vi "Ins_UARTWithBuffer.vi"(0 "COM":refnum<visa-resource-name>, 1 "Send":string, 3 "Timeout (ms)":u32=2000, 5 "Function":T1(ring)=enum."SendCompare", 9 "Baudrate":u32=921600, 11 "error in (no error)":errorcluster, 12 "REC":string) -> (6 "pass?":bool, 8 "ReceiveString":string, 10 "Return":string, 15 "error out":errorcluster)   [LabVIEW 2020, in "UART.lvlib"]
uses:
  UART.lvlib
  <vilib>/Instr/_visa.llb/VISA Set IO Buffer Mask.ctl
  75df8ced-9b69-4a5e-8517-458ef4cbff5d.vi
  <vilib>/Instr/_visa.llb/VISA Configure Serial Port (Instr).vi
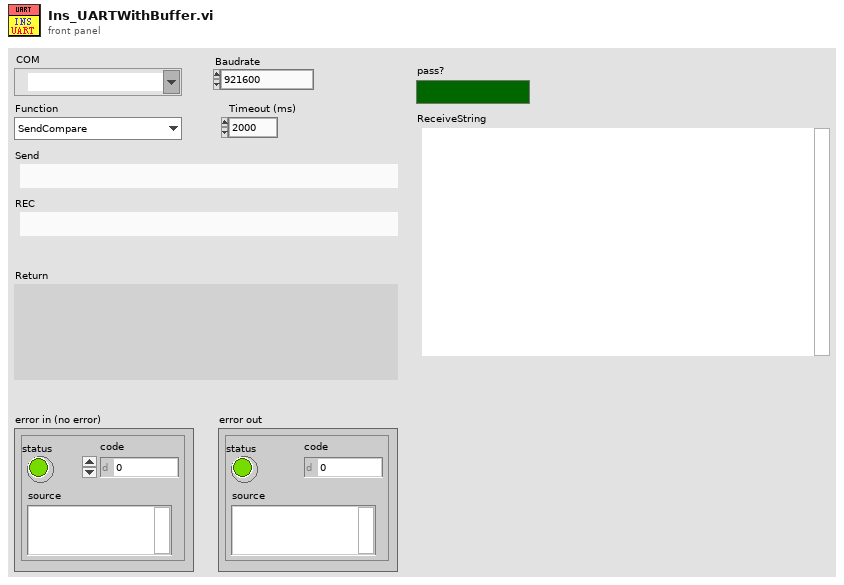
[diagram p1: front panel]
types:
  T1 = enum16{"Open", "Close", "Send", "Read", "SendWaitRead", "SendCompare", "ReadCompare"}
  T2 = typedef "VISA Set IO Buffer Mask.ctl" = u16
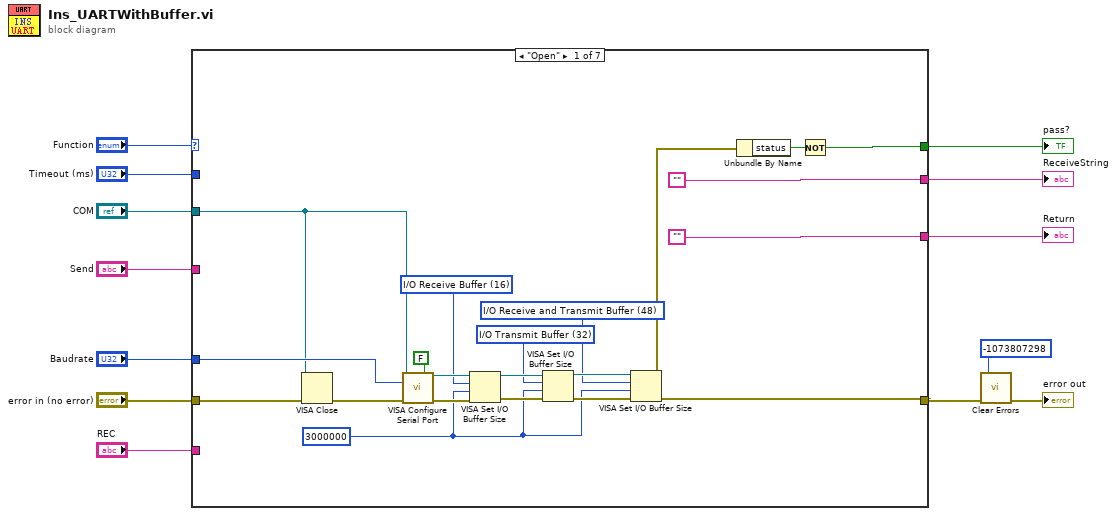
[diagram p0: block diagram]
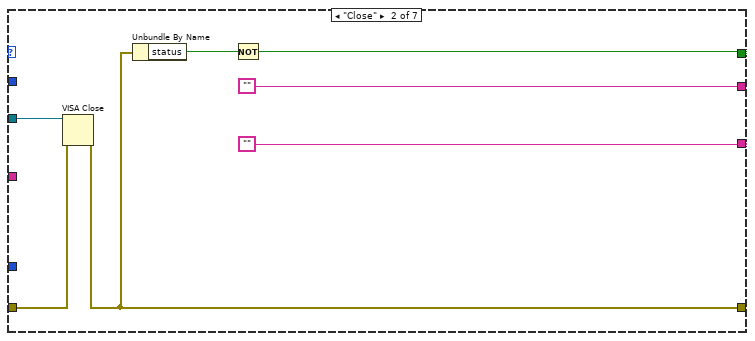
[diagram p2: hidden frame]
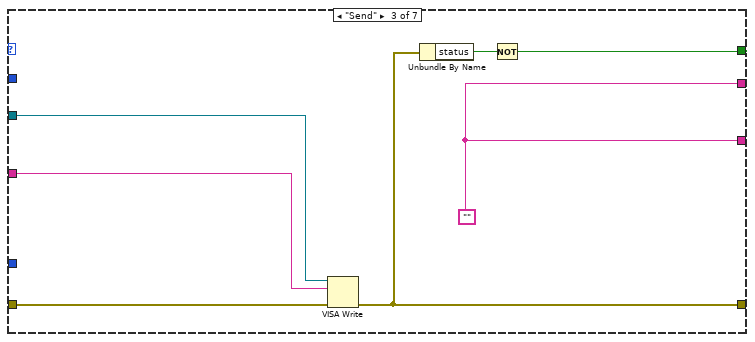
[diagram p3: hidden frame]
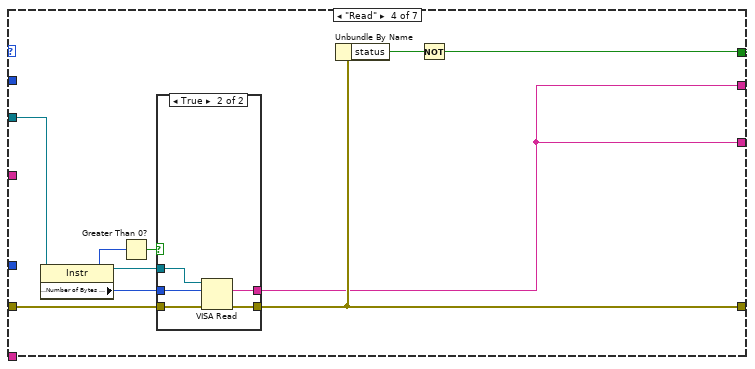
[diagram p4: hidden frame]
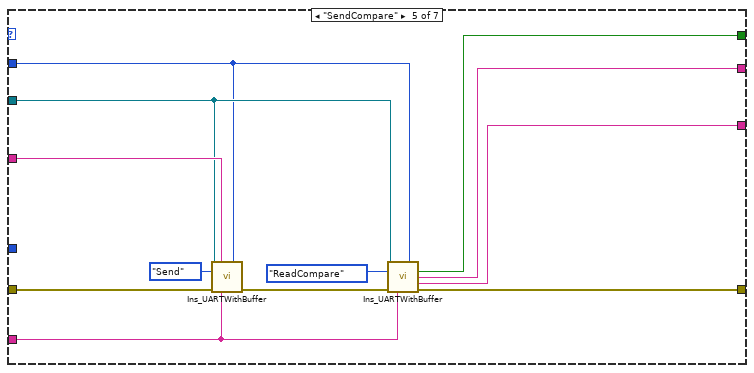
[diagram p6: hidden frame]
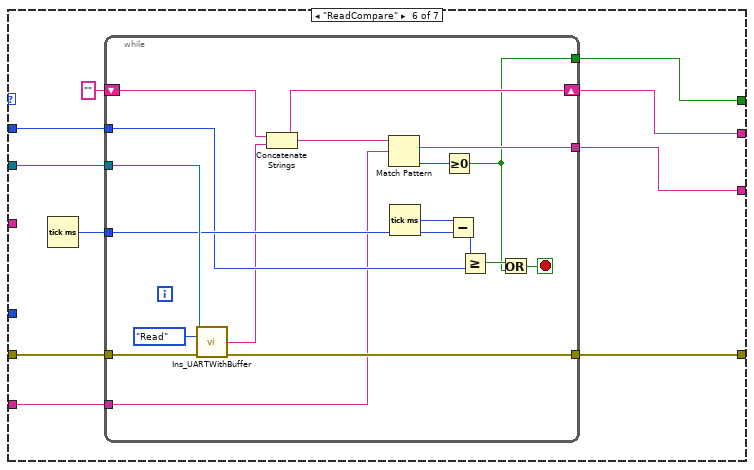
[diagram p7: hidden frame]
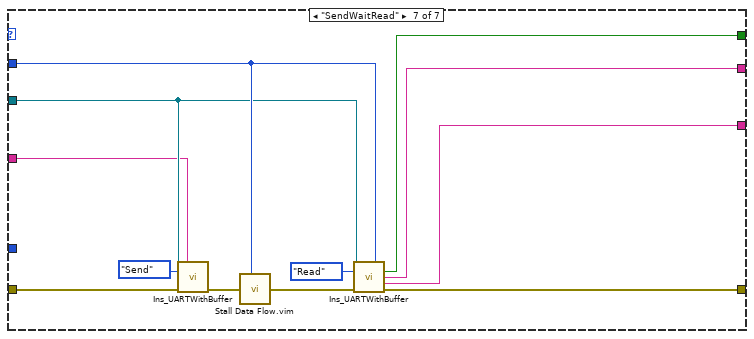
[diagram p8: hidden frame]
diagram:
  n1 = case shown="\"Open\"" "Function" {
    tunnel: "Send" -> [_ _ w41 _ w74 _ w104]
    tunnel: "error in (no error)" -> [w28 w37 w44 w52 w68 w83 w103]
    tunnel: [w14 w36 w45 w54 w73 w82 w112] -> w4
    tunnel: [w33 w39 w46 w55 w71 w75 w109] -> w13
    tunnel: ["" "" w42 w48 w70 w76 w111] -> w1
    tunnel: "COM" -> [w29 w38 w43 w53 w66 w84 w105]
    tunnel: "Baudrate" -> [w32 _ _ _ _ _ _]
    tunnel: "Timeout (ms)" -> [_ _ _ _ w64 w80 w107]
    tunnel: "REC" -> [_ _ _ _ w63 w81 _]
    tunnel: ["" "" w42 w48 w69 w77 w110] -> w2
    frame "Open" {
      w16 = T2 16 items=["I/O Receive Buffer"=16, "I/O Transmit Buffer"=32, "I/O Receive and Transmit Buffer"=48] ("Mask")
      w17 = T2 48 items=["I/O Receive Buffer"=16, "I/O Transmit Buffer"=32, "I/O Receive and Transmit Buffer"=48] ("Mask")
      w18 = T2 32 items=["I/O Receive Buffer"=16, "I/O Transmit Buffer"=32, "I/O Receive and Transmit Buffer"=48] ("Mask")
      w19 = u32 3000000 ("size (4096)")
      n2 = VISA Close(VISA resource name=w29, error in (no error)=w28) -> (error out=w27:errorcluster)
      n3 = call-poly "VISA Configure Serial Port"("VISA resource name"=w29, "Enable Termination\nChar (T)"=FALSE ("Enable Termination\nChar (T)"), "baud rate (9600)"=w32, "error in (no error)"=w27) -> ("VISA resource name out"=w24:refnum<visa-resource-name>, "error out"=w25:errorcluster)  [unwired: 4 in, 6 out]
      n4 = VISA Set I/O Buffer Size(VISA resource name=w24, mask (16)=w16, size (4096)=w19, error in (no error)=w25) -> (VISA resource name out=w23:refnum<visa-resource-name>, error out=w21:errorcluster)
      n5 = VISA Set I/O Buffer Size(VISA resource name=w23, mask (16)=w18, size (4096)=w19, error in (no error)=w21) -> (VISA resource name out=w22:refnum<visa-resource-name>, error out=w20:errorcluster)
      n6 = VISA Set I/O Buffer Size(VISA resource name=w22, mask (16)=w17, size (4096)=w19, error in (no error)=w20) -> (error out=w14:errorcluster)  [unwired: 1 out]
      n7 = Unbundle By Name(w14) -> ("status"=w15:bool)
      n8 = Not(x=w15) -> (.not. x?=w33:bool)
    }
    frame "Close" {
      n9 = VISA Close(VISA resource name=w38, error in (no error)=w37) -> (error out=w36:errorcluster)
      n10 = Unbundle By Name(w36) -> ("status"=w40:bool)
      n11 = Not(x=w40) -> (.not. x?=w39:bool)
    }
    frame "Send" {
      w42 = ""
      n12 = VISA Write(VISA resource name=w43, write buffer=w41, error in (no error)=w44) -> (error out=w45:errorcluster)  [unwired: 2 out]
      n13 = Unbundle By Name(w45) -> ("status"=w47:bool)
      n14 = Not(x=w47) -> (.not. x?=w46:bool)
    }
    frame "Read" {
      n15 = property class="Instr"(reference=w53) -> (reference out=w51:refnum<visa-resource-name>, "Serial Settings:Number of Bytes at Serial Port"=w50:u32)  [unwired: 1 in, 1 out]
      n16 = Greater Than 0?(x=w50) -> (x > 0?=w49:bool)
      n17 = case shown="True" w49 {
        tunnel: [w57 w62] -> w54
        tunnel: w52 -> [w57 w61]
        tunnel: w51 -> [_ w60]
        tunnel: [_ w59] -> w48
        tunnel: w50 -> [_ w58]
        frame False {
        }
        frame True {
          n18 = VISA Read(VISA resource name=w60, byte count=w58, error in (no error)=w61) -> (read buffer=w59:string, error out=w62:errorcluster)  [unwired: 2 out]
        }
      }
      n19 = Unbundle By Name(w54) -> ("status"=w56:bool)
      n20 = Not(x=w56) -> (.not. x?=w55:bool)
    }
    frame "SendCompare" {
      n21 = call "Ins_UARTWithBuffer.vi"("COM"=w66, "Send"=w74, "Timeout (ms)"=w64, "Function"=T1."Send", "error in (no error)"=w68, "REC"=w63) -> ("error out"=w67:errorcluster)  [unwired: 6 in, 3 out]
      n22 = call "Ins_UARTWithBuffer.vi"("COM"=w66, "Timeout (ms)"=w64, "Function"=T1."ReadCompare", "error in (no error)"=w67, "REC"=w63) -> ("pass?"=w71:bool, "ReceiveString"=w70:string, "Return"=w69:string, "error out"=w73:errorcluster)  [unwired: 7 in]
    }
    frame "ReadCompare" {
      n23 = Tick Count (ms)() -> (millisecond timer value=w79:u32)
      n24 = while {
        tunnel: w84 -> [w100]
        tunnel: w83 -> [w101]
        tunnel: [w98] -> w82
        tunnel: w81 -> [w91]
        tunnel: w80 -> [w94]
        tunnel: w79 -> [w97]
        shift-right: [w89] -> w76
        shift-left: "" ("ReceiveString") -> [w92]
        tunnel: [w90] -> w77
        tunnel: [w85] -> w75
        stop <- w87 stop-if-true
        n25 = call "Ins_UARTWithBuffer.vi"("COM"=w100, "Function"=T1."Read", "error in (no error)"=w101) -> ("ReceiveString"=w93:string, "error out"=w98:errorcluster)  [unwired: 9 in, 2 out]
        n26 = Concatenate Strings(w92, w93) -> (w89:string)
        n27 = Match Pattern(string=w89, regular expression=w91) -> (match substring=w90:string, offset past match=w88:i32)  [unwired: 1 in, 2 out]
        n28 = Tick Count (ms)() -> (millisecond timer value=w96:u32)
        n29 = Greater Or Equal To 0?(x=w88) -> (x >= 0?=w85:bool)
        n30 = Subtract(x=w96, y=w97) -> (x-y=w95:u32)
        n31 = Greater Or Equal?(x=w95, y=w94) -> (x >= y?=w86:bool)
        n32 = Or(x=w86, y=w85) -> (x .or. y?=w87:bool)
      }
    }
    frame "SendWaitRead" {
      n33 = call "Ins_UARTWithBuffer.vi"("COM"=w105, "Send"=w104, "Function"=T1."Send", "error in (no error)"=w103) -> ("error out"=w102:errorcluster)  [unwired: 8 in, 3 out]
      n34 = call "Stall Data Flow.vim"("value in"=w102, "milliseconds to wait"=w107) -> ("value out"=w108:errorcluster)  [unwired: 1 out]
      n35 = call "Ins_UARTWithBuffer.vi"("COM"=w105, "Timeout (ms)"=w107, "Function"=T1."Read", "error in (no error)"=w108) -> ("pass?"=w109:bool, "ReceiveString"=w111:string, "Return"=w110:string, "error out"=w112:errorcluster)  [unwired: 8 in]
    }
  }
  "pass?" <- w13
  "Return" <- w2
  "ReceiveString" <- w1
  n36 = call <vilib>:"Clear Errors.vi"("error in (no error)"=w4, "specific error code to clear (0: all)"=-1073807298) -> ("error out"=→"error out":errorcluster)  [unwired: 4 in, 1 out]
